vi "prompt_synthesis.vi"(8 "error in (no error)":errorcluster, 10 "search_results":T1[](array[typedef]), 11 "agent_simple_qa in":refnum<class "agent_simple_qa.lvclass">) -> (0 "error out":errorcluster, 2 "prompt_synthesiser":refnum<class "message_text.lvclass">, 3 "agent_simple_qa out":refnum<class "agent_simple_qa.lvclass">)   [LabVIEW 2020, in "agent_simple_qa.lvclass"]
uses:
  agent_simple_qa.lvclass
  vectorstore/abstract_vector_base/search result.ctl
  vectorstore/abstract_vector_base/vector.ctl
  models/message_text/message_text.lvclass
  models/message_text/create_text_message.vi
  vectorstore/abstract_vector_base/abstract_vector_base.lvclass
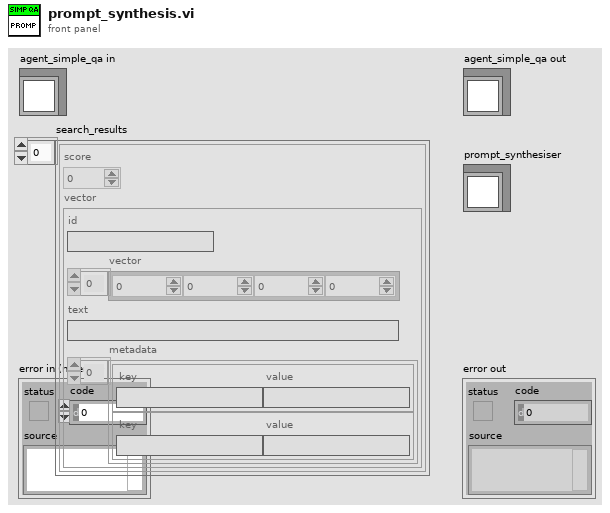
[diagram p1: front panel]
types:
  T1 = typedef "abstract_vector_base.lvclass/search result.ctl" = cluster{"score":dbl, "vector":T2}
  T2 = typedef "abstract_vector_base.lvclass/vector.ctl" = cluster{"id":string, "vector":dbl[], "text":string, "metadata":cluster{"key":string, "value":string}[]}
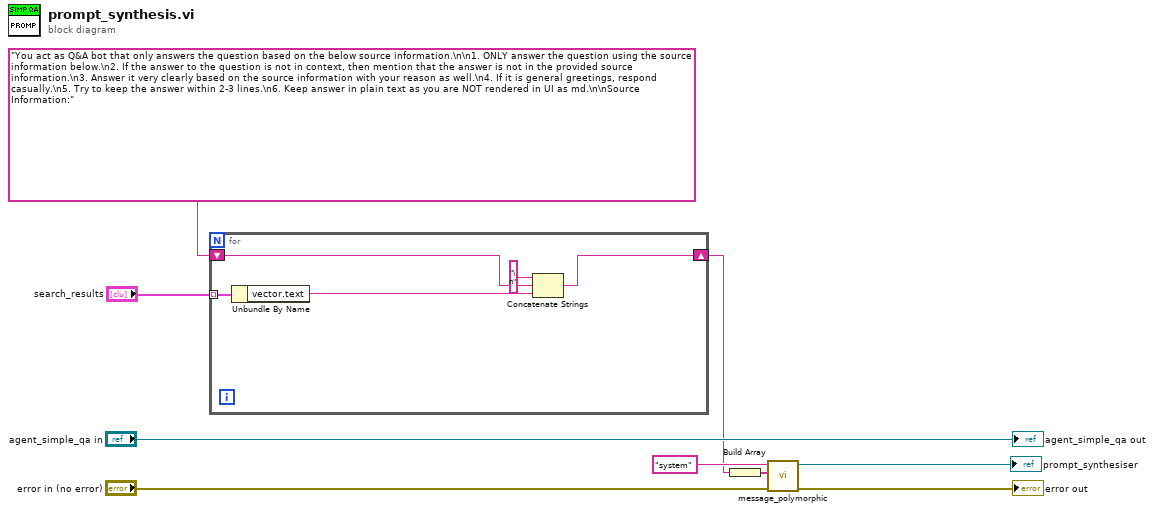
[diagram p0: block diagram]
diagram:
  n1 = for {
    tunnel: "search_results" -> [w14] mode=indexing
    shift-right: [w11] -> w2
    shift-left: "You act as Q&A bot that only answers the question based on the below source information.\n\n1. ONLY answer the question using the source information below.\n2. If the answer to the question is not in context, then mention that the answer is not in the provided source information.\n3. Answer it very clearly based on the source information with your reason as well.\n4. If it is general greetings, respond casually.\n5. Try to keep the answer within 2-3 lines.\n6. Keep answer in plain text as you are NOT rendered in UI as md.\n\nSource Information:" -> [w13]
    n2 = Unbundle By Name(w14) -> ("vector.text"=w12:string)
    n3 = Concatenate Strings("\n" ("string"), w13, w12) -> (w11:string)
  }
  n4 = Build Array(w2) -> (w5:string[])
  n5 = call-poly "message_polymorphic.vi"("error in (no error)"="error in (no error)", "content"=w5, "role"="system") -> ("error out"=→"error out":errorcluster, "message_text out"=→"prompt_synthesiser":refnum<class "message_text.lvclass">)  [unwired: 7 in]
  "agent_simple_qa out" <- "agent_simple_qa in"
